vi "Check_Data.vi"(0 "Vpp_0":dbl, 1 "Width_0":dbl, 2 "Setup_Time_0":dbl, 3 "Vpp_Array":dbl[](array[numeric]), 4 "Width Array":dbl[](array[numeric]), 5 "Setup_Time_Array":dbl[](array[numeric]), 6 "Percentage_Range":i32=5 min=5 max=50 step=5, 7 "file path (dialog if empty)":path, 8 "file path (dialog if empty) 2":path, 9 "Delay Line Number":i32, 11 "Delay Index":i32, 13 "error in 1":errorcluster) -> (19 "error in 2":errorcluster)   [LabVIEW 2009]
uses:
  <vilib>/Utility/file.llb/Write To Spreadsheet File (string).vi
  <vilib>/Analysis/NI_AALBase.lvlib
panel:
  in  "Delay_Value":dbl[](array[numeric])=[0.0, 0.25, 0.5, 0.75, 1.0, 1.25, 1.5, 1.75, 2.0, 2.25, 2.5, 2.75, 3.0, 3.25, 3.5, 3.75, 4.0, 4.25, 4.5, 4.75, 5.0, 5.25, 5.5, 5.75, 2.0, 2.25, 2.5, 2.75, 3.0, 3.25, 3.5, 3.75]
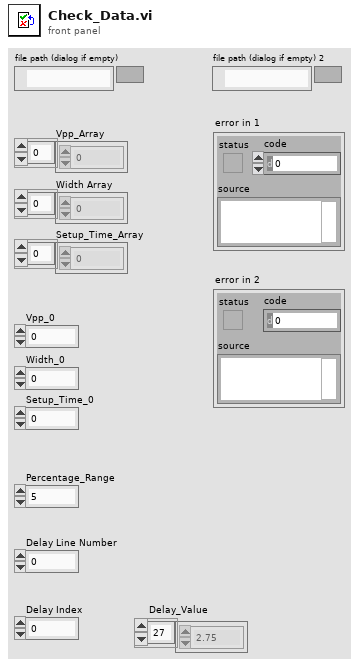
[diagram p1: front panel]
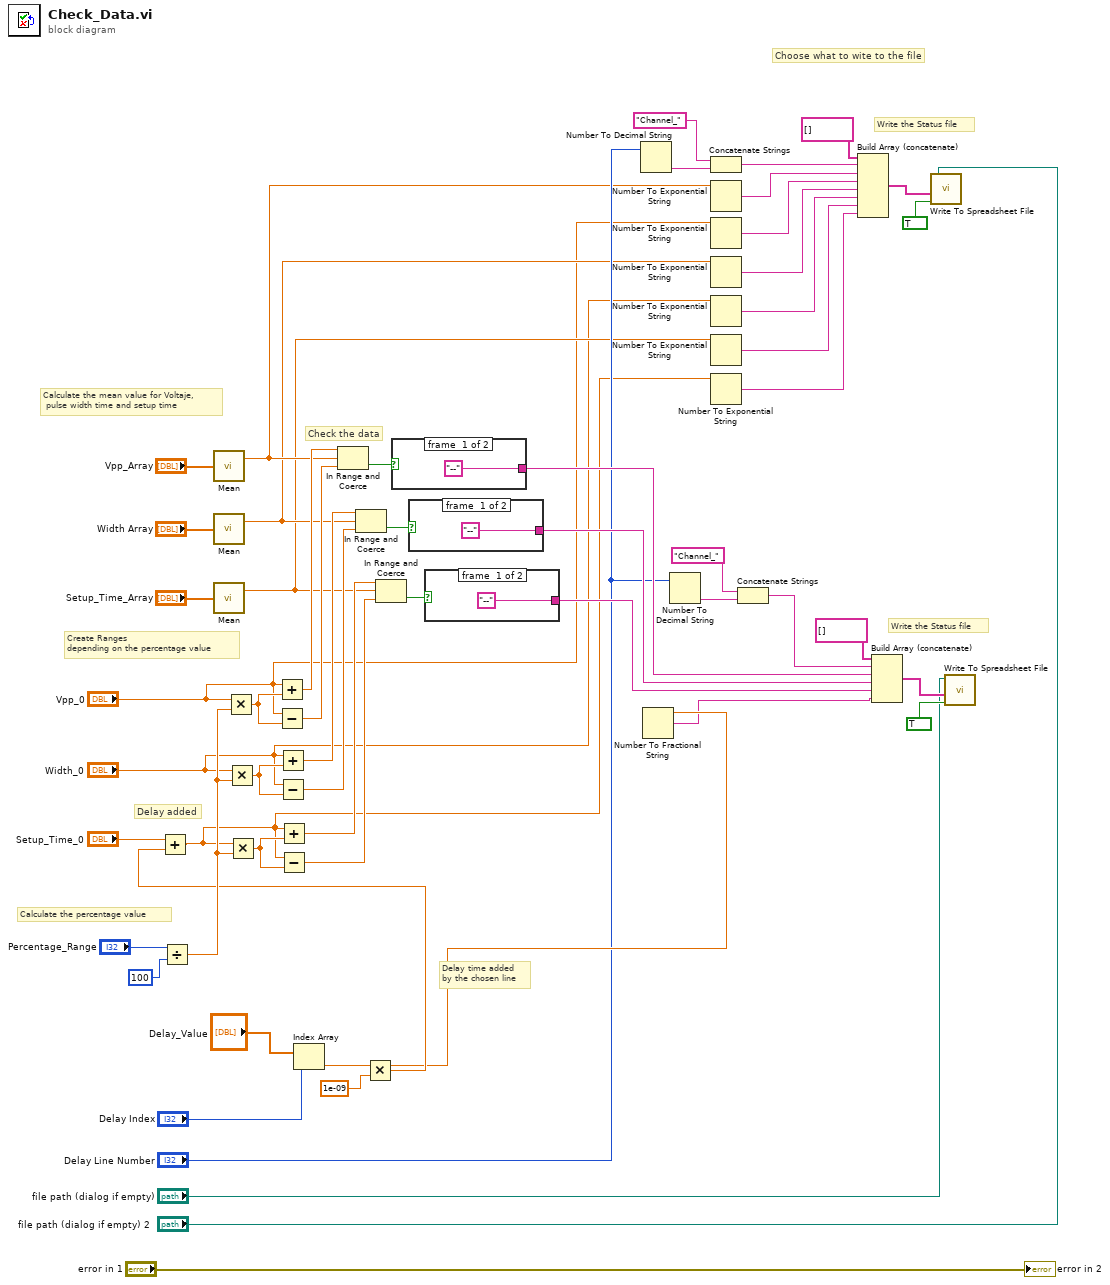
[diagram p0: block diagram]
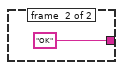
[diagram p2: hidden frame]
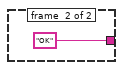
[diagram p3: hidden frame]
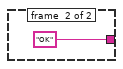
[diagram p4: hidden frame]
diagram:
  # "Write the Status file"
  # "Delay added"
  # "Delay time added \nby the chosen line"
  # "Write the Status file"
  # "Check the data"
  # "Choose what to wite to the file"
  # "Calculate the percentage value"
  # "Create Ranges\ndepending on the percentage value"
  # "Calculate the mean value for Voltaje,\n pulse width time and setup time"
  n1 = Divide(x="Percentage_Range", y=100) -> (x/y=w38:dbl)
  n2 = call <vilib>:"Mean.vi"("X"="Vpp_Array") -> ("mean"=w13:dbl)  [unwired: 1 out]
  n3 = call <vilib>:"Mean.vi"("X"="Width Array") -> ("mean"=w5:dbl)  [unwired: 1 out]
  n4 = call <vilib>:"Mean.vi"("X"="Setup_Time_Array") -> ("mean"=w4:dbl)  [unwired: 1 out]
  n5 = Multiply(x="Vpp_0", y=w38) -> (x*y=w51:dbl)
  n6 = Multiply(x="Width_0", y=w38) -> (x*y=w43:dbl)
  n7 = Add(x="Vpp_0", y=w51) -> (x+y=w50:dbl)
  n8 = Subtract(x="Vpp_0", y=w51) -> (x-y=w49:dbl)
  n9 = Add(x="Width_0", y=w43) -> (x+y=w42:dbl)
  n10 = Subtract(x="Width_0", y=w43) -> (x-y=w41:dbl)
  n11 = Index Array(array="Delay_Value", index="Delay Index") -> (element=w24:dbl)
  n12 = In Range and Coerce(upper limit=w50, x=w13, lower limit=w49) -> (In Range?=w48:bool)  [unwired: 1 out]
  n13 = In Range and Coerce(upper limit=w42, x=w5, lower limit=w41) -> (In Range?=w40:bool)  [unwired: 1 out]
  n14 = Multiply(x=w24, y=1e-09) -> (x*y=w28:dbl)
  n15 = Add(x="Setup_Time_0", y=w28) -> (x+y=w7:dbl)
  n16 = Multiply(x=w7, y=w38) -> (x*y=w39:dbl)
  n17 = Add(x=w7, y=w39) -> (x+y=w37:dbl)
  n18 = Subtract(x=w7, y=w39) -> (x-y=w36:dbl)
  n19 = In Range and Coerce(upper limit=w37, x=w4, lower limit=w36) -> (In Range?=w35:bool)  [unwired: 1 out]
  n20 = case shown="False" w48 {
    tunnel: ["--" "OK"] -> w32
    frame #0 {
    }
    frame #1 {
    }
  }
  n21 = case shown="False" w40 {
    tunnel: ["--" "OK"] -> w33
    frame #0 {
    }
    frame #1 {
    }
  }
  n22 = case shown="False" w35 {
    tunnel: ["--" "OK"] -> w34
    frame #0 {
    }
    frame #1 {
    }
  }
  n23 = Number To Decimal String(number="Delay Line Number") -> (decimal integer string=w17:string)  [unwired: 1 in]
  n24 = Number To Fractional String(number=w24) -> (F-format string=w22:string)  [unwired: 3 in]
  n25 = Number To Decimal String(number="Delay Line Number") -> (decimal integer string=w27:string)  [unwired: 1 in]
  n26 = Concatenate Strings("Channel_", w17) -> (w15:string)
  n27 = Number To Exponential String(number=w13) -> (E-format string=w12:string)  [unwired: 3 in]
  n28 = Number To Exponential String(number="Vpp_0") -> (E-format string=w11:string)  [unwired: 3 in]
  n29 = Number To Exponential String(number=w5) -> (E-format string=w10:string)  [unwired: 3 in]
  n30 = Number To Exponential String(number="Width_0") -> (E-format string=w8:string)  [unwired: 3 in]
  n31 = Number To Exponential String(number=w4) -> (E-format string=w1:string)  [unwired: 3 in]
  n32 = Number To Exponential String(number=w7) -> (E-format string=w6:string)  [unwired: 3 in]
  n33 = Concatenate Strings("Channel_", w27) -> (w23:string)
  n34 = Build Array (concatenate)(string[] [] ("array"), w15, w12, w11, w10, w8, w1, w6) -> (w19:string[])
  n35 = Build Array (concatenate)(string[] [] ("array"), w23, w32, w33, w34, w22) -> (w46:string[])
  n36 = call-poly <vilib>:"Write To Spreadsheet File.vi"("append to file? (new file:F)"=TRUE, "1D data"=w19, "file path (dialog if empty)"="file path (dialog if empty) 2") -> ()  [unwired: 5 in, 1 out]
  n37 = call-poly <vilib>:"Write To Spreadsheet File.vi"("append to file? (new file:F)"=TRUE, "1D data"=w46, "file path (dialog if empty)"="file path (dialog if empty)") -> ()  [unwired: 5 in, 1 out]
  "error in 2" <- "error in 1"
